vi "File Browser.vi"(11 "Shutdown Event":refnum<user-event>) -> ()   [LabVIEW 2019, in "User Interface.lvlib"]
doc: "File browser sub panel. Tracks are dragged and dropped from here to the DJ interface to load them.\n\n<b>Execution System:</b> User Interface"
uses:
  User Interface.lvlib
  Custom Graphics/Listbox.Browser.ctl
  <vilib>/Utility/sysdir.llb/System Directory Type.ctl
  Tree Browser/Tree Browser.lvlib
panel:
  in  "File List":T1=-1
  in  "Directory Tree":string(tree)
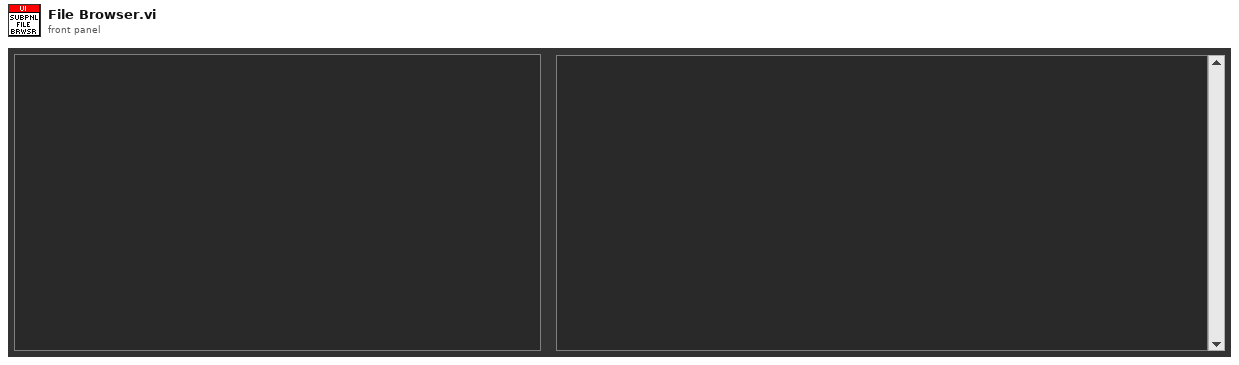
[diagram p1: front panel]
types:
  T1 = typedef "User Interface.lvlib/Listbox.Browser.ctl" = i32
  T2 = typedef "System Directory Type.ctl" = i32
  T3 = cluster{"data name":string, "drag data":variant}[]
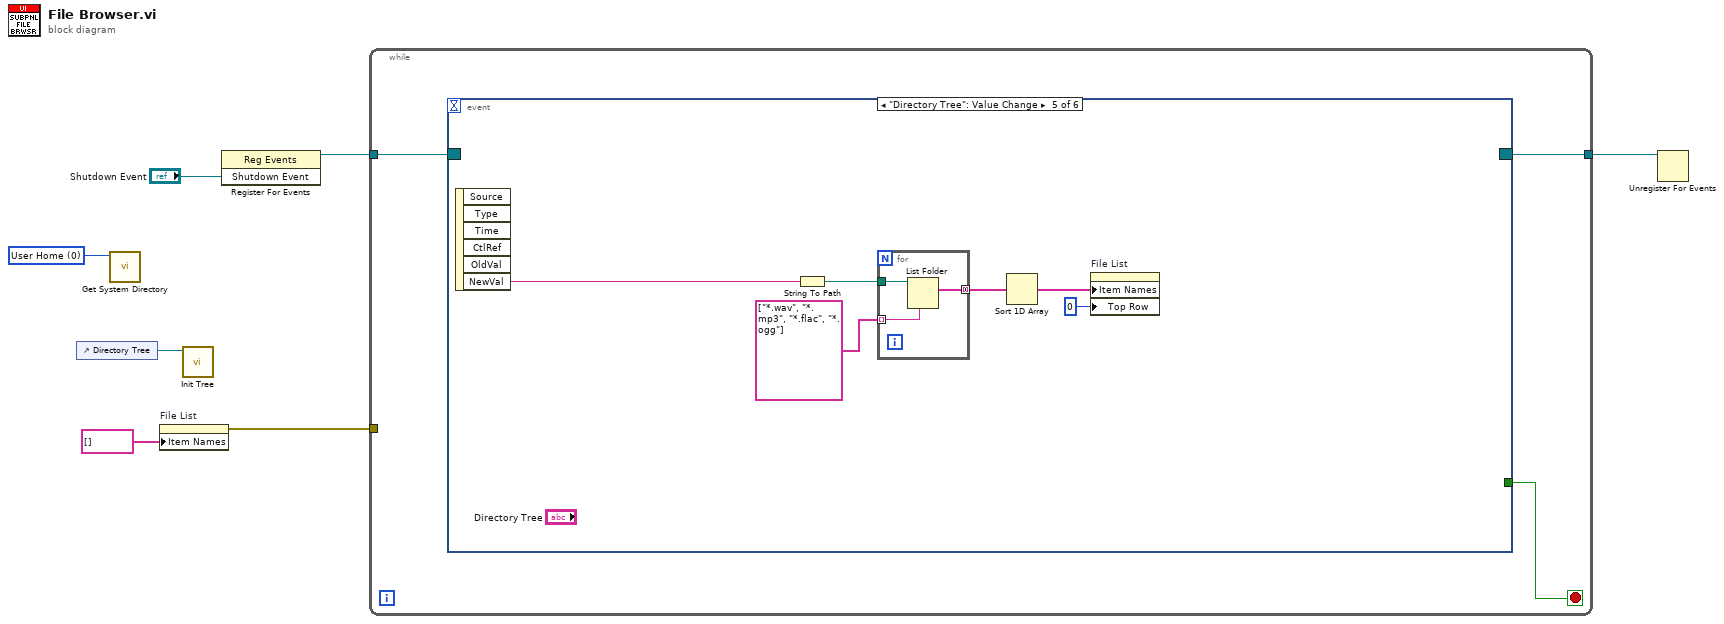
[diagram p0: block diagram]
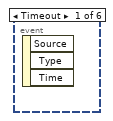
[diagram p2: hidden frame]
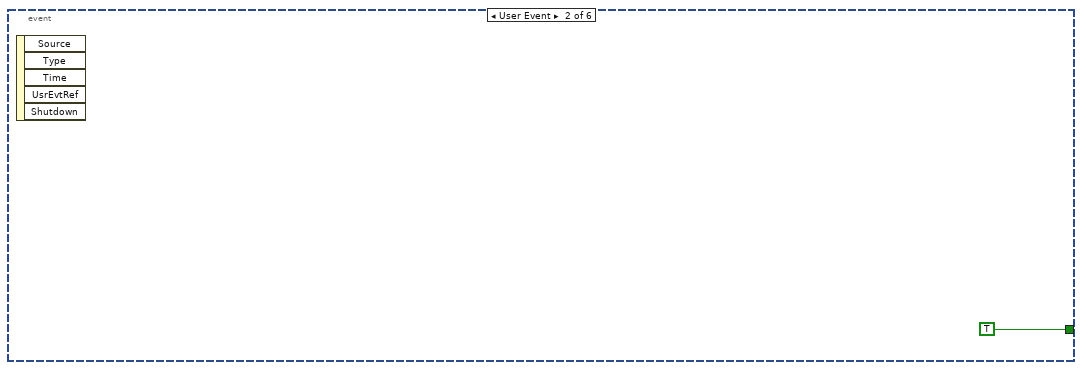
[diagram p3: hidden frame]
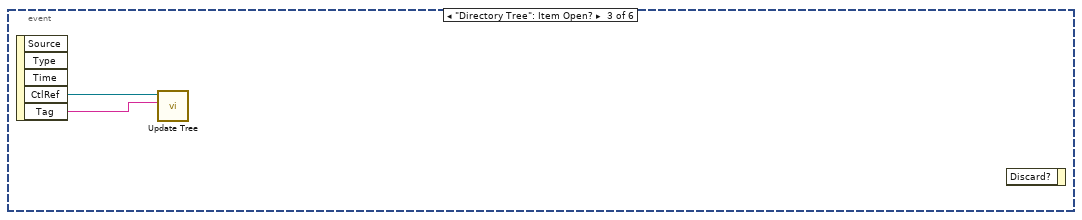
[diagram p4: hidden frame]
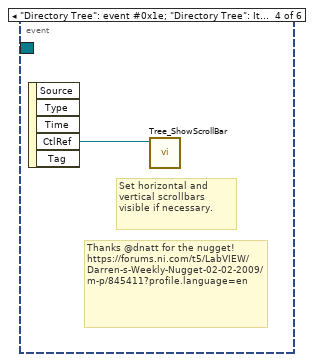
[diagram p5: hidden frame]
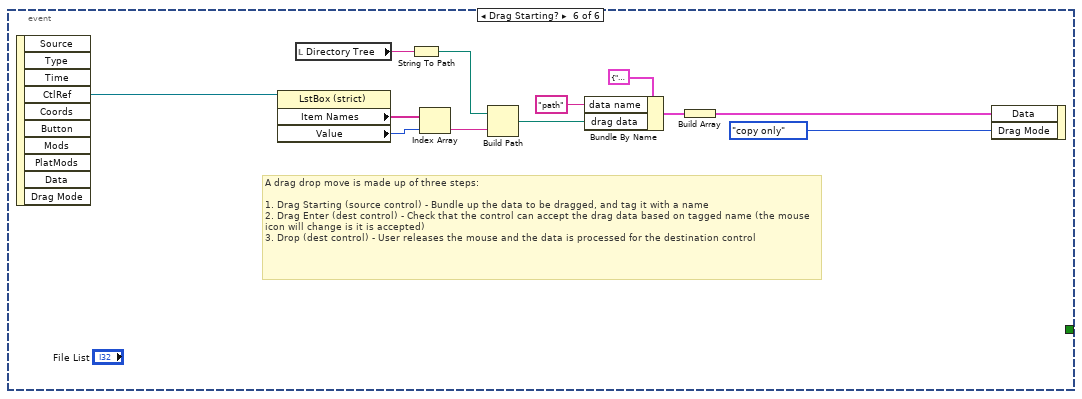
[diagram p6: hidden frame]
diagram:
  w7 = T2 0 items=["User Home"=0, "User Desktop"=1, "User Documents"=2, "User Application Data"=3, "User Preferences"=4, "User Temporary"=5, "Public Documents"=6, "Public Application Data"=7, "Public Preferences"=8, "Public Cache"=13, "System Core Libraries"=9, "System Installed Libraries"=10, "Application Files"=11, "Boot Volume Root"=12] ("system directory type")
  n1 = control-ref of="Directory Tree"() -> (w2:refnum<vi>)
  n2 = call <vilib>:"Get System Directory.vi"("system directory type"=w7) -> ()  [unwired: 10 in, 1 out]
  n3 = property on="File List" class="LstBox (strict)"("Item Names"=string[] []) -> (error out=w1:errorcluster)  [unwired: 2 in, 1 out]
  n4 = call "Init Tree.vi"("Tree In"=w2) -> ()  [unwired: 10 in, 1 out]
  n5 = register-events("Shutdown Event") -> (reference out=w4:refnum<event-registration>)  [unwired: 2 in, 1 out]
  n6 = while {
    tunnel: w4 -> [w10]
    tunnel: [w8] -> w3
    tunnel: w1 -> [_]
    stop <- w9 stop-if-true
    n7 = event shown="[4] \"Directory Tree\": Value Change" {
      selector: w10 -> [_ _ _ _ _ _]
      dyn-events: [_ _ _ _ _ _] -> w8
      timeout: _ -> [_ _ _ _ _ _]
      tunnel: [_ TRUE _ _ _ _] -> w9
      event Timeout {
        n8 = event-data() -> ()  [unwired: 1 in, 3 out]
      }
      event User Event {
        n9 = event-data() -> ()  [unwired: 1 in, 5 out]
      }
      event "Directory Tree": Item Open? {
        n10 = event-data() -> ("CtlRef"=w13:refnum<vi>, "Tag"=w12:string)  [unwired: 1 in, 3 out]
        n11 = call "Update Tree.vi"("Parent Tag"=w12, "Tree In"=w13) -> ()  [unwired: 9 in, 1 out]
        n12 = event-data() -> ()  [unwired: 2 in, 1 out]
      }
      event "Directory Tree": event #0x1e; "Directory Tree": Item Close {
        # "Thanks @dnatt for the nugget!\nhttps://forums.ni.com/t5/LabVIEW/Darren-s-Weekly-Nugget-02-02-2009/m-p/845411?profile.language=en"
        # "Set horizontal and vertical scrollbars visible if necessary."
        n13 = event-data() -> ("CtlRef"=w14:refnum<vi>)  [unwired: 1 in, 4 out]
        n14 = call <vilib>:"Tree_ShowScrollBar.vi"("Tree"=w14) -> ()  [unwired: 10 in, 1 out]
      }
      event "Directory Tree": Value Change {
        n15 = event-data() -> ("NewVal"=w16:string)  [unwired: 1 in, 5 out]
        n16 = String To Path(string=w16) -> (path=w15:path)
        n17 = for {
          tunnel: [w23] -> w19 mode=concatenating
          tunnel: w15 -> [w22]
          tunnel: string[] ["*.wav", "*.mp3", "*.flac", "*.ogg"] -> [w21] mode=indexing
          n18 = List Folder(path=w22, pattern=w21) -> (filenames=w23:string[])  [unwired: 2 in, 3 out]
        }
        n19 = Sort 1D Array(array=w19) -> (sorted array=w18:string[])
        n20 = property on="File List" class="LstBox (strict)"("Item Names"=w18, "Top Row"=0) -> ()  [unwired: 2 in, 2 out]
      }
      event Drag Starting? {
        # "A drag drop move is made up of three steps:\n\n1. Drag Starting (source control) - Bundle up the data to be dragged, and tag it with a name\n2. Drag Enter (dest control) - Check that the control can accept the drag data based on tagged name (the mouse icon will change is it is accepted)\n3. Drop (dest control) - User releases the mouse and the data is processed for the destination control"
        n21 = event-data() -> ("CtlRef"=w27:refnum<vi>)  [unwired: 1 in, 9 out]
        n22 = property class="LstBox (strict)"(reference=w27) -> ("Item Names"=w34:string[], "Value"=w33:i32)  [unwired: 1 in, 2 out]
        n23 = local read "Directory Tree"() -> (w35:string)
        n24 = String To Path(string=w35) -> (path=w24:path)
        n25 = Index Array(array=w34, index=w33) -> (element=w31:string)
        n26 = Build Path(base path=w24, name or relative path=w31) -> (appended path=w30:path)
        n27 = Bundle By Name(cluster=cluster{"data name":string, "drag data":variant} {"data name"="", "drag data"=variant}, "data name"="path", "drag data"=w30) -> (w28:cluster{"data name":string, "drag data":variant})
        n28 = Build Array(w28) -> (w25:T3)
        n29 = event-data("Data"=w25, "Drag Mode"=enum32{"copy or move", "copy only", "move only"}."copy only") -> ()  [unwired: 1 in, 1 out]
      }
    }
  }
  n30 = Unregister For Events(event registration refnum=w3) -> ()  [unwired: 1 in, 1 out]
